vi "CSU22 Device Engine.vi"(0 "XLight Notifier Name":string="CSU22", 11 "COM Port":string[](array[string])) -> ()   [LabVIEW 2020]
uses:
  Spinning Disk Type Defs/SD Actions.ctl
  Spinning Disk Type Defs/SD Notifer Data.ctl
  <vilib>/Instr/_visa.llb/VISA Configure Serial Port (Instr).vi
panel:
  in  "Home All":bool
  in  "Get All Positions":bool
  in  "Disk On":bool
  in  "Disk Position":i32=1 min=1 max=3
  in  "Dichroic":i32=1 min=1 max=5
  in  "Ex Ba Filter":i32=1 min=1 max=8
  out "Latest Error":errorcluster
  in  "Quit":bool
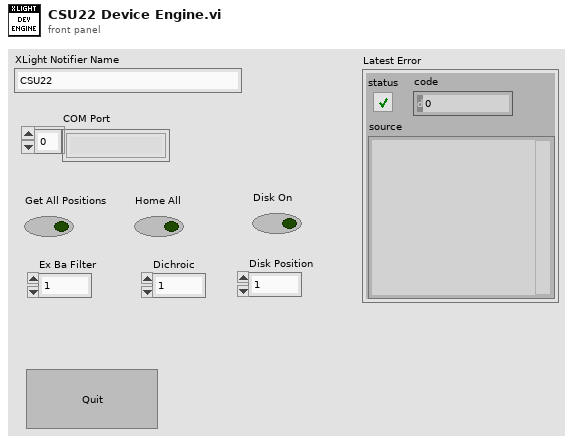
[diagram p1: front panel]
types:
  T1 = typedef "SD Notifer Data.ctl" = cluster{"Actions":T2, "Disk On?":bool, "Dichroic Pos.":i32, "Filter Wheel Pos.":i32, "Disk Pos.":i32, "Recived":bool, "Num Pos":i32[]}
  T2 = typedef "SD Actions.ctl" = enum16{"Status", "Get All Pos.", "Get Num. Pos.", "Home All", "Set Filter Wheel Pos.", "Set Disk Pos.", "Set Dichroic Pos.", "Disk On", "Disk Off", "Quit"}
  T3 = enum32{"Invalid", "Standard", "Closed", "Hidden", "Minimized", "Maximized"}
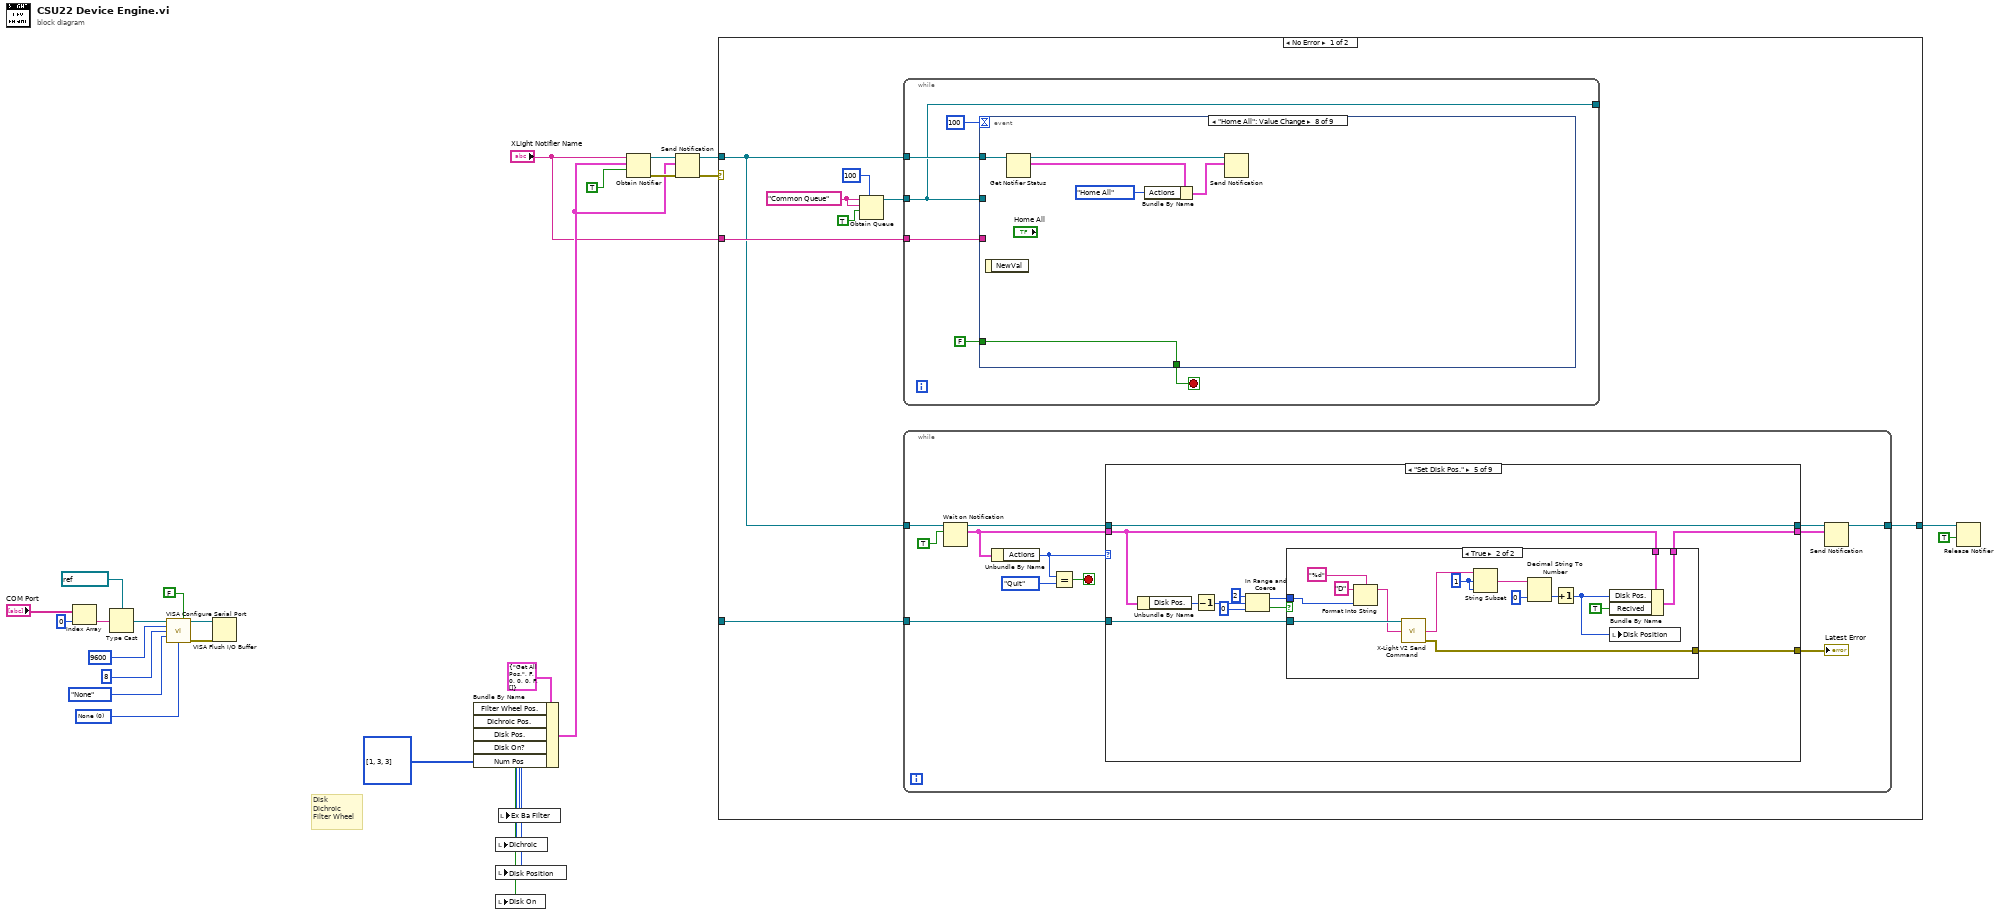
[diagram p0: block diagram]
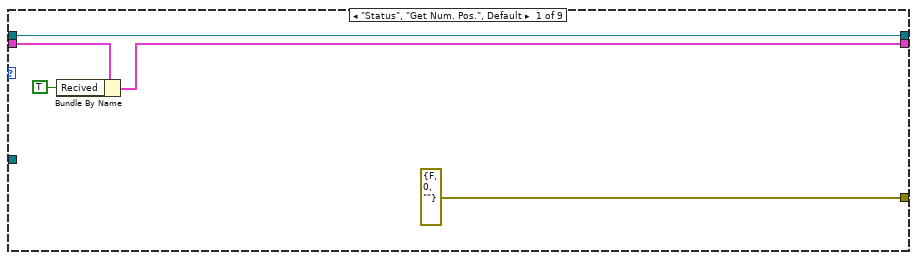
[diagram p2: hidden frame]
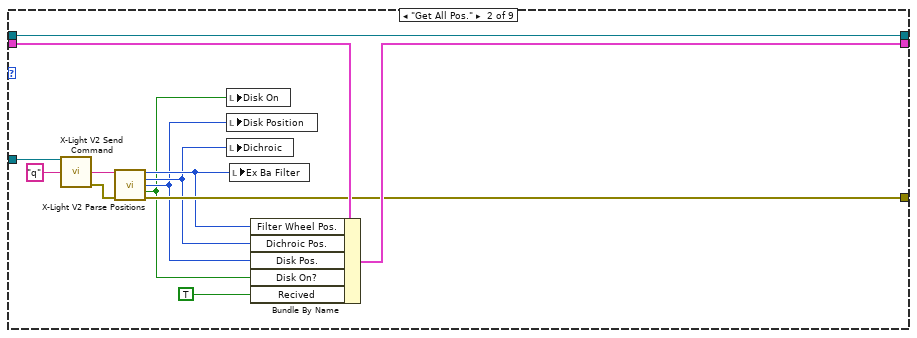
[diagram p3: hidden frame]
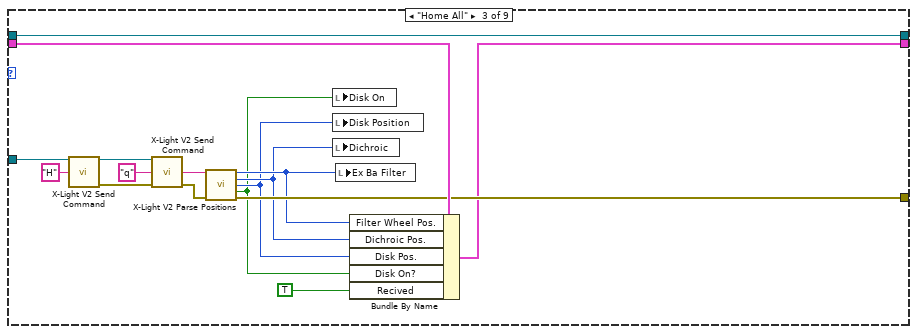
[diagram p4: hidden frame]
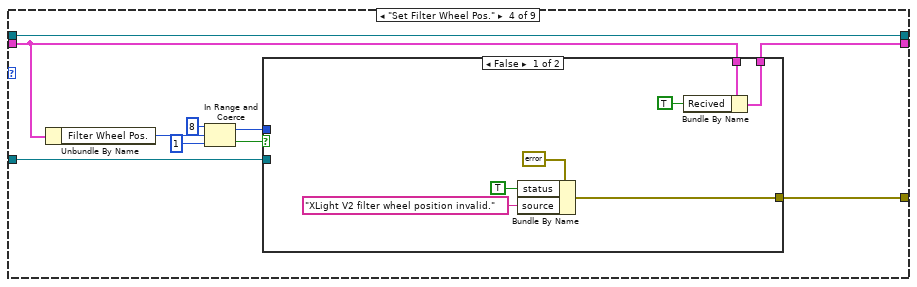
[diagram p5: hidden frame]
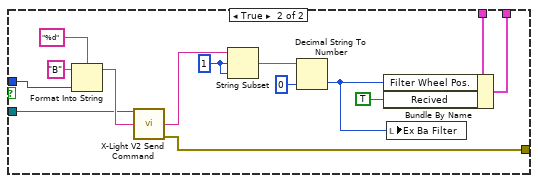
[diagram p6: hidden frame]
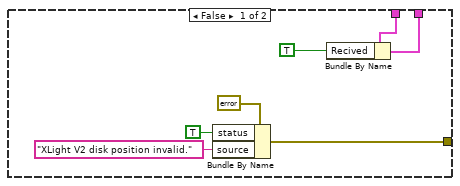
[diagram p7: hidden frame]
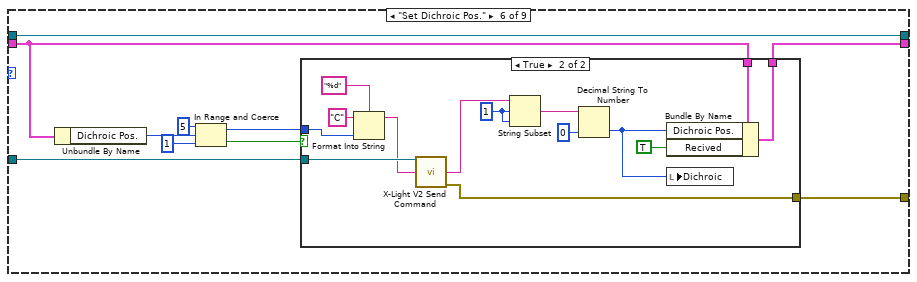
[diagram p8: hidden frame]
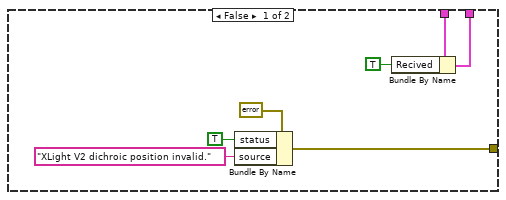
[diagram p9: hidden frame]
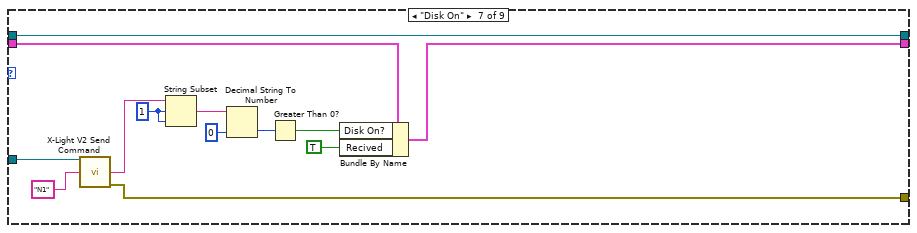
[diagram p10: hidden frame]
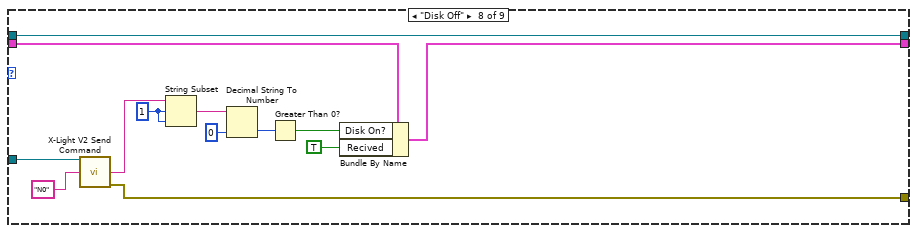
[diagram p11: hidden frame]
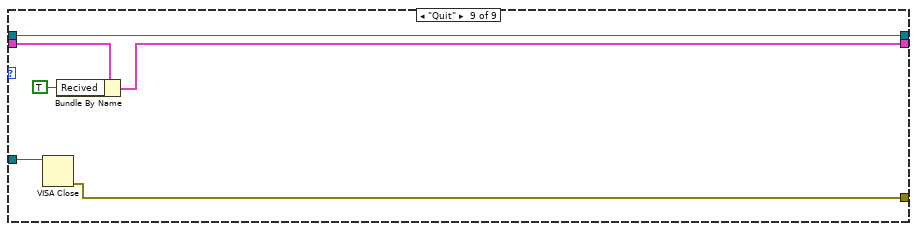
[diagram p12: hidden frame]
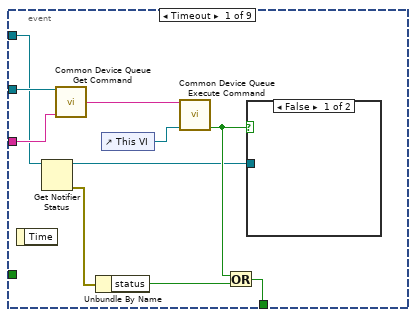
[diagram p13: hidden frame]
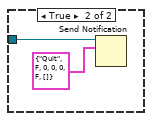
[diagram p14: hidden frame]
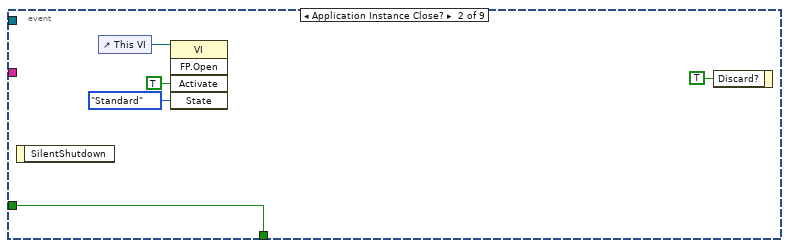
[diagram p15: hidden frame]
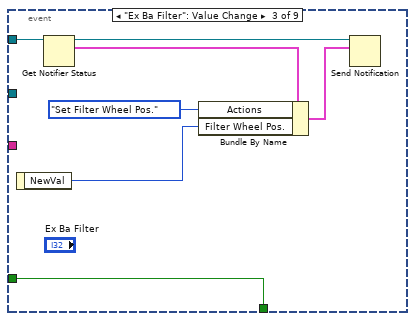
[diagram p16: hidden frame]
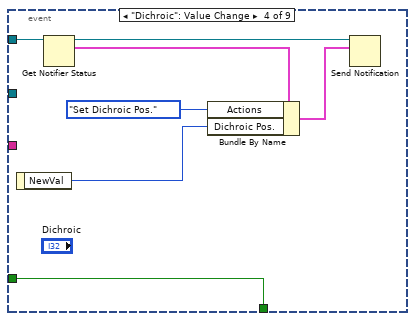
[diagram p17: hidden frame]
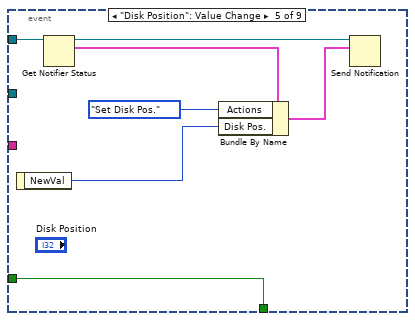
[diagram p18: hidden frame]
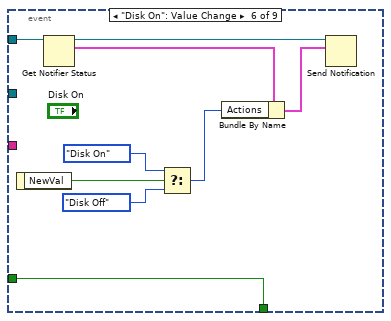
[diagram p19: hidden frame]
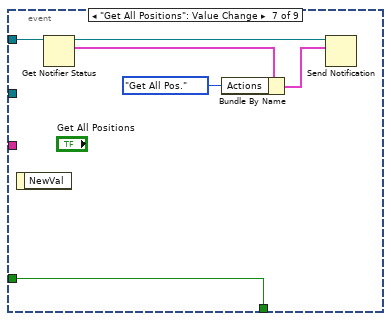
[diagram p20: hidden frame]
diagram:
  w4 = u16 0 items=["None", "XON/XOFF", "RTS/CTS", "XON/XOFF & RTS/CTS", "DTR/DSR", "XON/XOFF & DTR/DSR"] ("flow control (0:none)")
  # "Disk\nDichroic\nFilter Wheel"
  n1 = Index Array(array="COM Port", index=0) -> (element=w26:string)
  n2 = Type Cast(type=refnum<visa-resource-name> "COM5" ("VISA resource name"), x=w26) -> (*(type *) &x=w3:refnum<visa-resource-name>)
  n3 = call-poly "VISA Configure Serial Port"("VISA resource name"=w3, "Enable Termination\nChar (T)"=FALSE ("Enable Termination\nChar (T)"), "baud rate (9600)"=u32 9600, "data bits (8)"=u16 8, "parity (0:none)"=enum16{"None", "Odd", "Even", "Mark", "Space"}."None", "flow control (0:none)"=w4) -> ("VISA resource name out"=w2:refnum<visa-resource-name>, "error out"=w1:errorcluster)  [unwired: 8 in]
  n4 = VISA Flush I/O Buffer(VISA resource name=w2, error in (no error)=w1) -> ()  [unwired: 1 in, 2 out]
  n5 = Bundle By Name(cluster=T1 {"Actions"=enum."Get All Pos.", "Disk On?"=FALSE, "Dichroic Pos."=0, "Filter Wheel Pos."=0, "Disk Pos."=0, "Recived"=FALSE, "Num Pos"=[]} ("XLight Notifier Data"), "Num Pos"=i32[] [1, 3, 3]) -> (w21:T1, "Filter Wheel Pos."=w13:i32, "Dichroic Pos."=w12:i32, "Disk Pos."=w9:i32, "Disk On?"=w11:bool)
  n6 = local write "Dichroic"(w12) -> ()
  n7 = local write "Disk Position"(w9) -> ()
  n8 = local write "Disk On"(w11) -> ()
  n9 = local write "Ex Ba Filter"(w13) -> ()
  n10 = Obtain Notifier(name (unnamed)="XLight Notifier Name", notification data type=w21, create if not found? (T)=TRUE) -> (error in (no error)=w16:errorcluster, notifier out=w24:refnum<notifier>, error out=w23:errorcluster)  [unwired: 1 out]
  n11 = Send Notification(notification=w21, notifier=w24, error in (no error)=w23) -> (notifier out=w19:refnum<notifier>, error out=w20:errorcluster)
  n12 = case shown="No Error" w20 {
    tunnel: w19 -> [w31 w282]
    tunnel: [w32 _] -> w17
    tunnel: "XLight Notifier Name" -> [w37 _]
    tunnel: [w30 w282] -> w15
    frame No Error {
      w36 = "Common Queue" ("Unique Notifier Name")
      n13 = Obtain Queue(max queue size (-1, unlimited)=100, name (unnamed)=w36, element data type=w36, create if not found? (T)=TRUE) -> (queue out=w33:refnum<queue>)  [unwired: 1 in, 2 out]
      n14 = while {
        tunnel: w33 -> [w211]
        tunnel: w37 -> [w214]
        tunnel: w31 -> [w215]
        tunnel: [w211] -> _
        stop <- w213 stop-if-true
        # "ProScan 3 GUI and Common Queue Loop"
        n15 = event shown="[7] \"Home All\": Value Change" {
          selector: _ -> [_ _ _ _ _ _ _ _ _]
          dyn-events: _ -> [_ _ _ _ _ _ _ _ _]
          timeout: 100 -> [_ _ _ _ _ _ _ _ _]
          tunnel: w211 -> [w220 _ _ _ _ _ _ _ _]
          tunnel: w215 -> [w217 _ w239 w246 w253 w262 w268 w274 w280]
          tunnel: w214 -> [w219 _ _ _ _ _ _ _ _]
          tunnel: [w218 w233 w240 w247 w254 w263 w269 w275 w281] -> w213
          tunnel: FALSE -> [_ w233 w240 w247 w254 w263 w269 w275 _]
          event Timeout {
            n16 = event-data() -> ()  [unwired: 1 in, 1 out]
            n17 = Get Notifier Status(notifier=w217) -> (notifier out=w221:refnum<notifier>, error out=w226:errorcluster)  [unwired: 1 in, 3 out]
            n18 = call "Common Device Queue Get Command.vi"("Common Queue"=w220, "Notifier Name"=w219) -> ("Command"=w225:string)  [unwired: 12 in, 1 out]
            n19 = Unbundle By Name(w226) -> ("status"=w223:bool)
            n20 = control-ref of="This VI"() -> (w224:refnum<vi>)
            n21 = call "Common Device Queue Execute Command.vi"("Common Command"=w225, "VI Refnum"=w224) -> ("Quit?"=w222:bool)  [unwired: 12 in, 1 out]
            n22 = Or(x=w222, y=w223) -> (x .or. y?=w218:bool)
            n23 = case shown="False" w222 {
              tunnel: w221 -> [_ w228]
              frame False {
              }
              frame True {
                n24 = Send Notification(notification=T1 {"Actions"=enum."Quit", "Disk On?"=FALSE, "Dichroic Pos."=0, "Filter Wheel Pos."=0, "Disk Pos."=0, "Recived"=FALSE, "Num Pos"=[]} ("XLight Notifier Data"), notifier=w228) -> ()  [unwired: 1 in, 2 out]
              }
            }
          }
          event Application Instance Close? {
            n25 = event-data() -> ()  [unwired: 1 in, 1 out]
            n26 = control-ref of="This VI"() -> (w230:refnum<vi>)
            n27 = invoke class="VI" method="FP.Open"(reference=w230, "Activate"=TRUE ("Activate?"), "State"=T3."Standard") -> ()  [unwired: 2 in, 5 out]
            n28 = event-data("Discard?"=TRUE) -> ()  [unwired: 1 in, 1 out]
          }
          event "Ex Ba Filter": Value Change {
            n29 = event-data() -> ("NewVal"=w235:i32)  [unwired: 1 in]
            n30 = Get Notifier Status(notifier=w239) -> (notifier out=w238:refnum<notifier>, current notification=w237:T1)  [unwired: 1 in, 3 out]
            n31 = Bundle By Name(cluster=w237, "Actions"=SD_Actions."Set Filter Wheel Pos.", "Filter Wheel Pos."=w235) -> (w234:T1)
            n32 = Send Notification(notification=w234, notifier=w238) -> ()  [unwired: 1 in, 2 out]
          }
          event "Dichroic": Value Change {
            n33 = event-data() -> ("NewVal"=w242:i32)  [unwired: 1 in]
            n34 = Get Notifier Status(notifier=w246) -> (notifier out=w245:refnum<notifier>, current notification=w244:T1)  [unwired: 1 in, 3 out]
            n35 = Bundle By Name(cluster=w244, "Actions"=SD_Actions."Set Dichroic Pos.", "Dichroic Pos."=w242) -> (w241:T1)
            n36 = Send Notification(notification=w241, notifier=w245) -> ()  [unwired: 1 in, 2 out]
          }
          event "Disk Position": Value Change {
            n37 = event-data() -> ("NewVal"=w249:i32)  [unwired: 1 in]
            n38 = Get Notifier Status(notifier=w253) -> (notifier out=w252:refnum<notifier>, current notification=w251:T1)  [unwired: 1 in, 3 out]
            n39 = Bundle By Name(cluster=w251, "Actions"=SD_Actions."Set Disk Pos.", "Disk Pos."=w249) -> (w248:T1)
            n40 = Send Notification(notification=w248, notifier=w252) -> ()  [unwired: 1 in, 2 out]
          }
          event "Disk On": Value Change {
            n41 = event-data() -> ("NewVal"=w258:bool)  [unwired: 1 in]
            n42 = Get Notifier Status(notifier=w262) -> (notifier out=w261:refnum<notifier>, current notification=w260:T1)  [unwired: 1 in, 3 out]
            n43 = Select(t=SD_Actions."Disk On" ("Actions"), s=w258, f=SD_Actions."Disk Off" ("Actions")) -> (s? t:f=w255:T2)
            n44 = Bundle By Name(cluster=w260, "Actions"=w255) -> (w259:T1)
            n45 = Send Notification(notification=w259, notifier=w261) -> ()  [unwired: 1 in, 2 out]
          }
          event "Get All Positions": Value Change {
            n46 = event-data() -> ()  [unwired: 1 in, 1 out]
            n47 = Get Notifier Status(notifier=w268) -> (notifier out=w267:refnum<notifier>, current notification=w266:T1)  [unwired: 1 in, 3 out]
            n48 = Bundle By Name(cluster=w266, "Actions"=SD_Actions."Get All Pos.") -> (w265:T1)
            n49 = Send Notification(notification=w265, notifier=w267) -> ()  [unwired: 1 in, 2 out]
          }
          event "Home All": Value Change {
            n50 = event-data() -> ()  [unwired: 1 in, 1 out]
            n51 = Get Notifier Status(notifier=w274) -> (notifier out=w273:refnum<notifier>, current notification=w272:T1)  [unwired: 1 in, 3 out]
            n52 = Bundle By Name(cluster=w272, "Actions"=SD_Actions."Home All") -> (w271:T1)
            n53 = Send Notification(notification=w271, notifier=w273) -> ()  [unwired: 1 in, 2 out]
          }
          event "Quit": Value Change {
            n54 = event-data() -> ("NewVal"=w281:bool)  [unwired: 1 in]
            n55 = Get Notifier Status(notifier=w280) -> (notifier out=w277:refnum<notifier>, current notification=w279:T1)  [unwired: 1 in, 3 out]
            n56 = Bundle By Name(cluster=w279, "Actions"=SD_Actions."Quit") -> (w276:T1)
            n57 = Send Notification(notification=w276, notifier=w277) -> ()  [unwired: 1 in, 2 out]
          }
        }
      }
      n58 = while {
        tunnel: w32 -> [w40]
        tunnel: w31 -> [w49]
        tunnel: [w38] -> w30
        stop <- w46 stop-if-true
        n59 = Wait on Notification(notifier=w49, ignore previous (F)=TRUE) -> (notifier out=w44:refnum<notifier>, notification=w43:T1)  [unwired: 2 in, 2 out]
        n60 = Unbundle By Name(w43) -> ("Actions"=w45:T2)
        n61 = Equal?(x=w45, y=SD_Actions."Quit") -> (x = y?=w46:bool)
        n62 = case shown="\"Set Disk Pos.\"" w45 {
          tunnel: w44 -> [w54 w63 w72 w93 w125 w157 w191 w204 w210]
          tunnel: w43 -> [w53 w62 w76 w91 w122 w154 w188 w201 w209]
          tunnel: [w54 w63 w72 w93 w125 w157 w191 w204 w210] -> w42
          tunnel: [w51 w60 w73 w90 w121 w153 w182 w195 w207] -> w41
          tunnel: w40 -> [_ w64 w83 w86 w124 w156 w190 w203 w206]
          tunnel: [errorcluster {"status"=FALSE, "code"=0, "source"=""} ("Error Out") w59 w74 w92 w123 w155 w189 w202 w205] -> w39
          frame "Status", "Get Num. Pos.", Default {
            n63 = Bundle By Name(cluster=w53, "Recived"=TRUE) -> (w51:T1)
          }
          frame "Get All Pos." {
            n64 = call "X-Light V2 Send Command.vi"("VISA Resource"=w64, "Command"="q") -> ("Reply"=w66:string, "Error Out"=w65:errorcluster)  [unwired: 11 in, 1 out]
            n65 = call "X-Light V2 Parse Positions.vi"("Recived Reply"=w66, "Error In"=w65) -> ("Filter Wheel"=w58:i32, "Dichroic"=w57:i32, "Disk"=w56:i32, "Disk On"=w55:bool, "Error Out"=w59:errorcluster)  [unwired: 9 in]
            n66 = local write "Disk On"(w55) -> ()
            n67 = local write "Disk Position"(w56) -> ()
            n68 = local write "Dichroic"(w57) -> ()
            n69 = local write "Ex Ba Filter"(w58) -> ()
            n70 = Bundle By Name(cluster=w62, "Filter Wheel Pos."=w58, "Dichroic Pos."=w57, "Disk Pos."=w56, "Disk On?"=w55, "Recived"=TRUE) -> (w60:T1)
          }
          frame "Home All" {
            n71 = call "X-Light V2 Send Command.vi"("VISA Resource"=w83, "Command"="H") -> ("VISA Resource Out"=w78:refnum<visa-resource-name>, "Error Out"=w77:errorcluster)  [unwired: 11 in, 1 out]
            n72 = call "X-Light V2 Send Command.vi"("VISA Resource"=w78, "Command"="q", "Error In"=w77) -> ("Reply"=w80:string, "Error Out"=w79:errorcluster)  [unwired: 10 in, 1 out]
            n73 = call "X-Light V2 Parse Positions.vi"("Recived Reply"=w80, "Error In"=w79) -> ("Filter Wheel"=w71:i32, "Dichroic"=w70:i32, "Disk"=w69:i32, "Disk On"=w68:bool, "Error Out"=w74:errorcluster)  [unwired: 9 in]
            n74 = local write "Disk On"(w68) -> ()
            n75 = local write "Disk Position"(w69) -> ()
            n76 = local write "Dichroic"(w70) -> ()
            n77 = local write "Ex Ba Filter"(w71) -> ()
            n78 = Bundle By Name(cluster=w76, "Filter Wheel Pos."=w71, "Dichroic Pos."=w70, "Disk Pos."=w69, "Disk On?"=w68, "Recived"=TRUE) -> (w73:T1)
          }
          frame "Set Filter Wheel Pos." {
            n79 = Unbundle By Name(w91) -> ("Filter Wheel Pos."=w87:i32)
            n80 = In Range and Coerce(upper limit=8, x=w87, lower limit=1) -> (coerced(x)=w84:i32, In Range?=w85:bool)
            n81 = case shown="False" w85 {
              tunnel: [w97 w114] -> w92
              tunnel: w91 -> [w95 w110]
              tunnel: [w94 w104] -> w90
              tunnel: w86 -> [_ w103]
              tunnel: w84 -> [_ w102]
              frame False {
                n82 = Bundle By Name(cluster=errorcluster {"status"=FALSE, "code"=0, "source"=""} ("Error Out"), "status"=TRUE, "source"="XLight V2 filter wheel position invalid.") -> (w97:errorcluster)
                n83 = Bundle By Name(cluster=w95, "Recived"=TRUE) -> (w94:T1)
              }
              frame True {
                w107 = 1 ("offset (0)")
                n84 = Format Into String(format string="%d", initial string="B", w102) -> (resulting string=w111:string)  [unwired: 1 in, 1 out]
                n85 = call "X-Light V2 Send Command.vi"("VISA Resource"=w103, "Command"=w111) -> ("Reply"=w108:string, "Error Out"=w114:errorcluster)  [unwired: 11 in, 1 out]
                n86 = String Subset(string=w108, offset (0)=w107, length (rest)=w107) -> (substring=w106:string)
                n87 = Decimal String To Number(string=w106, default (0L)=0 ("default (0 I32)")) -> (number=w101:i32)  [unwired: 1 in, 1 out]
                n88 = Bundle By Name(cluster=w110, "Filter Wheel Pos."=w101, "Recived"=TRUE) -> (w104:T1)
                n89 = local write "Ex Ba Filter"(w101) -> ()
              }
            }
          }
          frame "Set Disk Pos." {
            n90 = Unbundle By Name(w122) -> ("Disk Pos."=w120:i32)
            n91 = Decrement(x=w120) -> (x-1=w115:i32)
            n92 = In Range and Coerce(upper limit=2, x=w115, lower limit=0) -> (coerced(x)=w116:i32, In Range?=w117:bool)
            n93 = case shown="True" w117 {
              tunnel: w124 -> [_ w147]
              tunnel: [w126 w146] -> w123
              tunnel: w122 -> [w131 w142]
              tunnel: [w130 w136] -> w121
              tunnel: w116 -> [_ w135]
              frame False {
                n94 = Bundle By Name(cluster=errorcluster {"status"=FALSE, "code"=0, "source"=""} ("Error Out"), "status"=TRUE, "source"="XLight V2 disk position invalid.") -> (w126:errorcluster)
                n95 = Bundle By Name(cluster=w131, "Recived"=TRUE) -> (w130:T1)
              }
              frame True {
                w139 = 1 ("offset (0)")
                n96 = Format Into String(format string="%d", initial string="D", w135) -> (resulting string=w143:string)  [unwired: 1 in, 1 out]
                n97 = call "X-Light V2 Send Command.vi"("VISA Resource"=w147, "Command"=w143) -> ("Reply"=w140:string, "Error Out"=w146:errorcluster)  [unwired: 11 in, 1 out]
                n98 = String Subset(string=w140, offset (0)=w139, length (rest)=w139) -> (substring=w138:string)
                n99 = Decimal String To Number(string=w138, default (0L)=0 ("default (0 I32)")) -> (number=w134:i32)  [unwired: 1 in, 1 out]
                n100 = Increment(x=w134) -> (x+1=w133:i32)
                n101 = Bundle By Name(cluster=w142, "Disk Pos."=w133, "Recived"=TRUE) -> (w136:T1)
                n102 = local write "Disk Position"(w133) -> ()
              }
            }
          }
          frame "Set Dichroic Pos." {
            n103 = Unbundle By Name(w154) -> ("Dichroic Pos."=w152:i32)
            n104 = In Range and Coerce(upper limit=5, x=w152, lower limit=1) -> (coerced(x)=w150:i32, In Range?=w151:bool)
            n105 = case shown="True" w151 {
              tunnel: w156 -> [_ w178]
              tunnel: [w161 w177] -> w155
              tunnel: w150 -> [_ w176]
              tunnel: w154 -> [w159 w172]
              tunnel: [w158 w166] -> w153
              frame False {
                n106 = Bundle By Name(cluster=errorcluster {"status"=FALSE, "code"=0, "source"=""} ("Error Out"), "status"=TRUE, "source"="XLight V2 dichroic position invalid.") -> (w161:errorcluster)
                n107 = Bundle By Name(cluster=w159, "Recived"=TRUE) -> (w158:T1)
              }
              frame True {
                w169 = 1 ("offset (0)")
                n108 = Format Into String(format string="%d", initial string="C", w176) -> (resulting string=w173:string)  [unwired: 1 in, 1 out]
                n109 = call "X-Light V2 Send Command.vi"("VISA Resource"=w178, "Command"=w173) -> ("Reply"=w170:string, "Error Out"=w177:errorcluster)  [unwired: 11 in, 1 out]
                n110 = String Subset(string=w170, offset (0)=w169, length (rest)=w169) -> (substring=w168:string)
                n111 = Decimal String To Number(string=w168, default (0L)=0 ("default (0 I32)")) -> (number=w165:i32)  [unwired: 1 in, 1 out]
                n112 = Bundle By Name(cluster=w172, "Dichroic Pos."=w165, "Recived"=TRUE) -> (w166:T1)
                n113 = local write "Dichroic"(w165) -> ()
              }
            }
          }
          frame "Disk On" {
            w185 = 1 ("offset (0)")
            n114 = call "X-Light V2 Send Command.vi"("VISA Resource"=w190, "Command"="N1" ("initial string")) -> ("Reply"=w186:string, "Error Out"=w189:errorcluster)  [unwired: 11 in, 1 out]
            n115 = String Subset(string=w186, offset (0)=w185, length (rest)=w185) -> (substring=w184:string)
            n116 = Decimal String To Number(string=w184, default (0L)=0 ("default (0 I32)")) -> (number=w181:i32)  [unwired: 1 in, 1 out]
            n117 = Greater Than 0?(x=w181) -> (x > 0?=w180:bool)
            n118 = Bundle By Name(cluster=w188, "Disk On?"=w180, "Recived"=TRUE) -> (w182:T1)
          }
          frame "Disk Off" {
            w198 = 1 ("offset (0)")
            n119 = call "X-Light V2 Send Command.vi"("VISA Resource"=w203, "Command"="N0" ("initial string")) -> ("Reply"=w199:string, "Error Out"=w202:errorcluster)  [unwired: 11 in, 1 out]
            n120 = String Subset(string=w199, offset (0)=w198, length (rest)=w198) -> (substring=w197:string)
            n121 = Decimal String To Number(string=w197, default (0L)=0 ("default (0 I32)")) -> (number=w194:i32)  [unwired: 1 in, 1 out]
            n122 = Greater Than 0?(x=w194) -> (x > 0?=w193:bool)
            n123 = Bundle By Name(cluster=w201, "Disk On?"=w193, "Recived"=TRUE) -> (w195:T1)
          }
          frame "Quit" {
            n124 = VISA Close(VISA resource name=w206) -> (error out=w205:errorcluster)  [unwired: 1 in]
            n125 = Bundle By Name(cluster=w209, "Recived"=TRUE) -> (w207:T1)
          }
        }
        "Latest Error" <- w39
        n126 = Send Notification(notification=w41, notifier=w42) -> (notifier out=w38:refnum<notifier>)  [unwired: 1 in, 1 out]
      }
    }
    frame Error {
    }
  }
  n127 = Release Notifier(notifier=w15, force destroy? (F)=TRUE) -> ()  [unwired: 1 in, 3 out]
